vi "Read Key Values.vi"(8 "error in":errorcluster, 11 "Config in":refnum<class "Config.lvclass">) -> (0 "error out":errorcluster, 3 "Config out":refnum<class "Config.lvclass">)   [LabVIEW 2023, in "Config.lvlib" / "Config.lvclass"]
uses:
  Config.lvclass
  Config.lvclass/Config.ctl
  <vilib>/Utility/config.llb/Read Key (String).vi
  <vilib>/Utility/config.llb/NI_LVConfig.lvlib
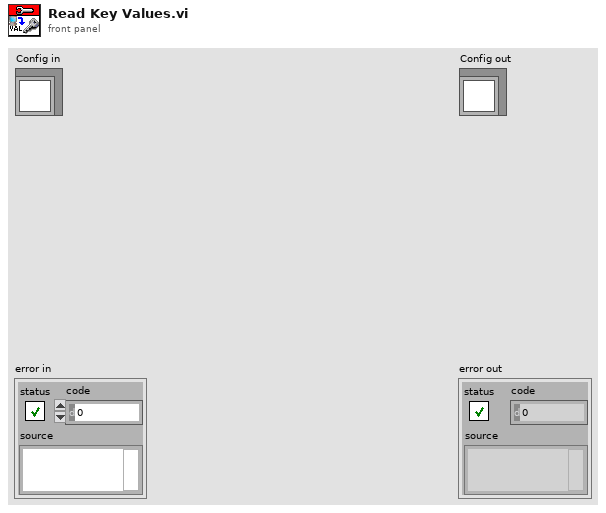
[diagram p1: front panel]
types:
  T1 = typedef "NI_LVConfig.lvlib/Config Data RefNum.ctl" = refnum<k1>
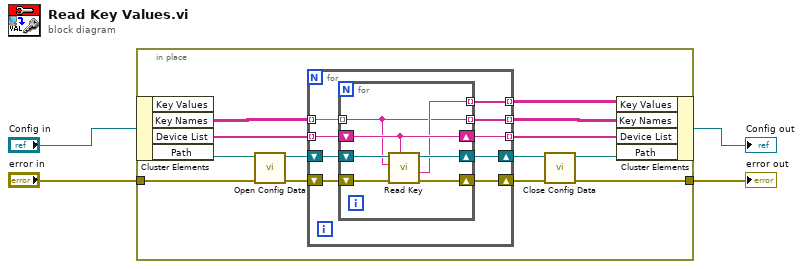
[diagram p0: block diagram]
diagram:
  n1 = in-place {
    in-place-border: "error in" -> [w11]
    in-place-border: [w10] -> w1
    n2 = in-place-cluster #1("Config in") -> ("Key Names"=w6:string[][], "Device List"=w9:string[], "Path"=w17:path)  [unwired: 1 out]
    n3 = call <vilib>:"Open Config Data.vi"("error in (no error)"=w11, "configuration file path"=w17) -> ("error out"=w15:errorcluster, "refnum"=w16:T1)  [unwired: 7 in, 1 out]
    n4 = for {
      shift-right: [w23] -> w14
      shift-left: w16 -> [w25]
      shift-right: [w22] -> w13
      shift-left: w15 -> [w24]
      tunnel: w9 -> [w21] mode=indexing
      tunnel: [w21] -> w8 mode=indexing
      tunnel: [w19] -> w7 mode=indexing
      tunnel: w6 -> [w20] mode=indexing
      tunnel: [w18] -> w5 mode=indexing
      n5 = for {
        shift-right: [w30] -> w23
        shift-left: w25 -> [w32]
        shift-right: [w29] -> w22
        shift-left: w24 -> [w31]
        shift-right: [w28] -> _
        shift-left: w21 -> [w28]
        tunnel: w20 -> [w26] mode=indexing
        tunnel: [w26] -> w19 mode=indexing
        tunnel: [w27] -> w18 mode=indexing
        n6 = call-poly <vilib>:"Read Key.vi"("section"=w28, "error in (no error)"=w31, "key"=w26, "refnum"=w32) -> ("error out"=w29:errorcluster, "value"=w27:string, "refnum out"=w30:T1)  [unwired: 4 in, 1 out]
      }
    }
    n7 = call <vilib>:"Close Config Data.vi"("error in (no error)"=w13, "refnum"=w14) -> ("error out"=w10:errorcluster, "file path"=w12:path)  [unwired: 8 in]
    n8 = in-place-cluster #1("Key Values"=w5, "Key Names"=w7, "Device List"=w8, "Path"=w12) -> (→"Config out":refnum<class "Config.lvclass">)
  }
  "error out" <- w1
